vi "crd_fitTau.vi"(11 "Channel A in":T1) -> (2 "tau (us)":dbl, 3 "Decay":dbl[](array[numeric]))   [LabVIEW 2011]
uses:
  <vilib>/Analysis/NI_AALPro.lvlib
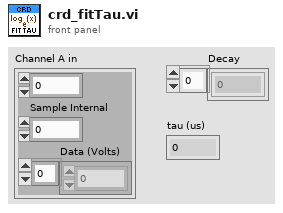
[diagram p1: front panel]
types:
  T1 = cluster{i32, "Sample Internal":sgl, "Data (Volts)":dbl[]}
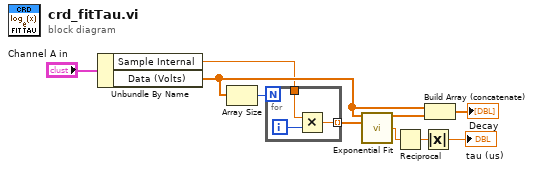
[diagram p0: block diagram]
diagram:
  n1 = Unbundle By Name("Channel A in") -> ("Sample Internal"=w9:sgl, "Data (Volts)"=w10:dbl[])
  n2 = Array Size(array=w10) -> (size(s)=w8:i32)
  n3 = for {
    N: w8 -> [_]
    tunnel: [w12] -> w2 mode=indexing
    tunnel: w9 -> [w11]
    i -> [w13]
    n4 = Multiply(x=w11, y=w13) -> (x*y=w12:sgl)
  }
  n5 = call <vilib>:"Exponential Fit.vi"("Y"=w10, "X"=w2) -> ("Best Exponential Fit"=w4:dbl[], "damping"=w5:dbl)  [unwired: 8 in, 4 out]
  n6 = Reciprocal(x=w5) -> (1/x=w6:dbl)
  n7 = Absolute Value(x=w6) -> (abs(x)=→"tau (us)":dbl)
  n8 = Build Array (concatenate)(w10, w4) -> (→"Decay":dbl[])
